vi "Clear TDC Measurement Valid.vi"(8 "error in":errorcluster, 11 "FPGA VI Reference In":T1) -> (0 "error out":errorcluster, 1 "tdc measurement":u16, 2 "measurement valid":bool, 3 "FPGA VI Reference Out":T1)   [LabVIEW 2011, in "FlexRIO Host Library (User).lvlib"]
uses:
  FlexRIO Host Library (User).lvlib
  <vilib>/rvi/interface/nirviReadWriteControl/nirviReadWriteControl.xnode
  Session/FPGA Session Ref.ctl
  Zeiss Acquisition Demo/FPGA Bitfiles/FlexRIODigitizer_FPGABoard_Acquire_Rev2.lvbitx
  <vilib>/rvi/errors/niLvFpgaMergeErrorWithErrorCode.vi
  <vilib>/rvi/errors/niLvFpgaAdjustHostInterfaceError.vi
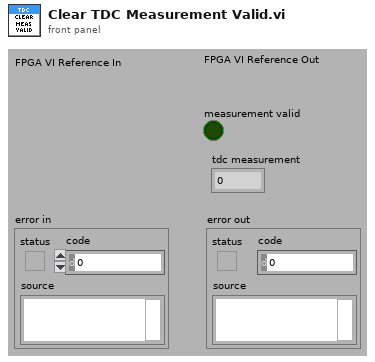
[diagram p1: front panel]
types:
  T1 = typedef "FlexRIO Host.lvlib/FPGA Session Ref.ctl" = refnum<k20>
  T2 = cluster{"clear meas valid":bool, "take a measurement":bool}
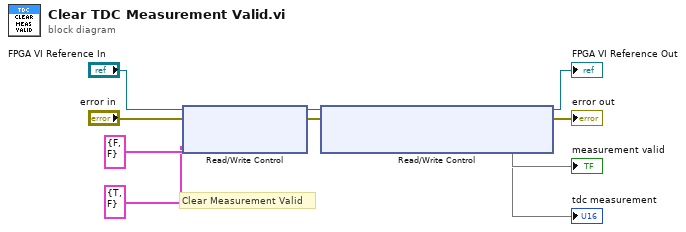
[diagram p0: block diagram]
diagram:
  # "Clear Measurement Valid"
  n1 = xnode "Read/Write Control"("FPGA VI Reference In"="FPGA VI Reference In", "error in"="error in", "TDC Control Signals"=T2 {"clear meas valid"=FALSE, "take a measurement"=FALSE}, "TDC Control Signals"=T2 {"clear meas valid"=TRUE, "take a measurement"=FALSE}) -> ("FPGA VI Reference Out"=w8:T1, "error out"=w7:errorcluster)
  n2 = xnode "Read/Write Control"("FPGA VI Reference In"=w8, "error in"=w7) -> ("FPGA VI Reference Out"=→"FPGA VI Reference Out":T1, "error out"=→"error out":errorcluster, "TDC Measurement.measurement is valid"=→"measurement valid", "TDC Measurement.tdc measurement"=→"tdc measurement")
